vi "UHR-Fleezers Control (host) - 11.9.vi"() -> ()   [LabVIEW 2014] (continued)
        n2874 = Array Subset(array=w4167, index (col)=0 ("index"), length (col)=w4156) -> (w4166:dbl[][])  [unwired: 2 in]
        n2875 = Array Subset(array=w4167, index (col)=w4156) -> (w4164:dbl[][])  [unwired: 3 in]
        n2876 = Array Subset(array=w4241, index (col)=0 ("index"), length (col)=w4156) -> (w4240:dbl[][])  [unwired: 2 in]
        n2877 = Array Subset(array=w4241, index (col)=w4156) -> (w4238:dbl[][])  [unwired: 3 in]
        n2878 = Array Subset(array=w4224, index (col)=0 ("index"), length (col)=w4156) -> (w4229:dbl[][])  [unwired: 2 in]
        n2879 = Array Subset(array=w4224, index (col)=w4156) -> (w4227:dbl[][])  [unwired: 3 in]
        n2880 = for {
          tunnel: w4236 -> [w4278] mode=indexing
          tunnel: [w4277] -> w4235 mode=indexing
          workers-P: _ -> [_]
          n2881 = Reverse 1D Array(array=w4278) -> (reversed array=w4277:dbl[])
        }
        n2882 = for {
          tunnel: w4222 -> [w4274] mode=indexing
          tunnel: [w4273] -> w4221 mode=indexing
          workers-P: _ -> [_]
          n2883 = Reverse 1D Array(array=w4274) -> (reversed array=w4273:dbl[])
        }
        n2884 = for {
          tunnel: w4166 -> [w4272] mode=indexing
          tunnel: [w4271] -> w4165 mode=indexing
          workers-P: _ -> [_]
          n2885 = Reverse 1D Array(array=w4272) -> (reversed array=w4271:dbl[])
        }
        n2886 = for {
          tunnel: w4240 -> [w4280] mode=indexing
          tunnel: [w4279] -> w4239 mode=indexing
          workers-P: _ -> [_]
          n2887 = Reverse 1D Array(array=w4280) -> (reversed array=w4279:dbl[])
        }
        n2888 = for {
          tunnel: w4229 -> [w4276] mode=indexing
          tunnel: [w4275] -> w4228 mode=indexing
          workers-P: _ -> [_]
          n2889 = Reverse 1D Array(array=w4276) -> (reversed array=w4275:dbl[])
        }
        n2890 = Index Array(array=w4241, index (row)=0) -> (element=→"Waveform Graph":dbl[])  [unwired: 1 in]
        n2891 = Add(x=w4235, y=w4234) -> (x+y=w4233:dbl[][])
        n2892 = Add(x=w4221, y=w4220) -> (x+y=w4219:dbl[][])
        n2893 = Add(x=w4165, y=w4164) -> (x+y=w4149:dbl[][])
        n2894 = Add(x=w4239, y=w4238) -> (x+y=w4213:dbl[][])
        n2895 = Add(x=w4228, y=w4227) -> (x+y=w4226:dbl[][])
        n2896 = Divide(x=w4219, y=2) -> (x/y=w4217:dbl[][])
        n2897 = Divide(x=w4233, y=2) -> (x/y=w4178:dbl[][])
        n2898 = Divide(x=w4226, y=2) -> (x/y=w4180:dbl[][])
        n2899 = To Single Precision Float(number=w4213) -> (single precision float=w4212:sgl[][])
        n2900 = Transpose 2D Array(2D array=w4217) -> (transposed array=→"Data map":dbl[][])
        n2901 = To Single Precision Float(number=w4149) -> (single precision float=w4153:sgl[][])
        n2902 = To Single Precision Float(number=w4178) -> (single precision float=w4184:sgl[][])
        n2903 = To Single Precision Float(number=w4180) -> (single precision float=w4181:sgl[][])
        n2904 = call "IMAQ ArrayToImage"("Image Pixels (Float)"=w4212, "Image"=w4146) -> ("Image Out"=w4215:T2)  [unwired: 8 in, 1 out]
        n2905 = call "IMAQ ArrayToImage"("Image Pixels (Float)"=w4153, "Image"=w4145) -> ("Image Out"=w4155:T2)  [unwired: 8 in, 1 out]
        n2906 = call "IMAQ ArrayToImage"("Image Pixels (Float)"=w4184, "Image"=w4144) -> ("Image Out"=w4186:T2)  [unwired: 8 in, 1 out]
        n2907 = call "IMAQ ArrayToImage"("Image Pixels (Float)"=w4181, "Image"=w4143) -> ("Image Out"=w4183:T2)  [unwired: 8 in, 1 out]
        n2908 = call "IMAQ Symmetry"("Type of Symmetry"=w4214, "Image Src"=w4215) -> ("Image Dst Out"=w4210:T2)  [unwired: 3 in, 1 out]
        n2909 = call "IMAQ Symmetry"("Type of Symmetry"=w4154, "Image Src"=w4155) -> ("Image Dst Out"=w4151:T2)  [unwired: 3 in, 1 out]
        n2910 = call "IMAQ Symmetry"("Type of Symmetry"=w4185, "Image Src"=w4186) -> ("Image Dst Out"=→"Detection Laser X":T2)  [unwired: 3 in, 1 out]
        n2911 = call "IMAQ Symmetry"("Type of Symmetry"=w4182, "Image Src"=w4183) -> ("Image Dst Out"=→"Detection Laser Y":T2)  [unwired: 3 in, 1 out]
        n2912 = call "IMAQ Set Simple Calibration"("Calibration Axis Info"=T36 {"Origin Pixel"={"X"=0.0, "Y"=0.0}, "Angle Relative to Horizontal (deg)"=0.0, "Axis Reference"=0}, "Grid Descriptor"=T37 {"X Step"=0.3, "Y Step"=0.3, "Unit"=enum."Undefined"}, "Image"=w4210) -> ("Calibrated Image"=→"APD 1":T2)  [unwired: 7 in, 1 out]
        n2913 = call "IMAQ Set Simple Calibration"("Calibration Axis Info"=T36 {"Origin Pixel"={"X"=0.0, "Y"=0.0}, "Angle Relative to Horizontal (deg)"=0.0, "Axis Reference"=0}, "Grid Descriptor"=T37 {"X Step"=0.3, "Y Step"=0.3, "Unit"=enum."Undefined"}, "Image"=w4151) -> ("Calibrated Image"=→"APD 2":T2)  [unwired: 7 in, 1 out]
      }
    }
    n2914 = Subtract(x=w3595, y="APD 2 Offset") -> (x-y=w3592:waveform(dbl))
    n2915 = Subtract(x=w3597, y="APD 1 Offset") -> (x-y=w3593:waveform(dbl))
    n2916 = Index Array(array=w3612, index=3) -> (element=w3672:waveform(dbl))
    n2917 = Index Array(array=w3612, index=6) -> (element=w3669:waveform(dbl))
    n2918 = Build Array(w3593, w3592) -> (→"APD Chart":waveform(dbl)[])
    n2919 = Array Size(array=w3663) -> (size(s)=w3716:i32)
    n2920 = call <vilib>:"Std Deviation and Variance.vi"("X"=w3605) -> ("standard deviation"=w3604:dbl)  [unwired: 1 in, 2 out]
    n2921 = Add Array Elements(numeric array=w3605) -> (sum=w3607:u32)
    n2922 = Add Array Elements(numeric array=w3663) -> (sum=w3726:u32)
    n2923 = call <vilib>:"Std Deviation and Variance.vi"("X"=w3663) -> ("standard deviation"=w3662:dbl)  [unwired: 1 in, 2 out]
    n2924 = Divide(x="T1 offset_x (mV)", y=1000.0) -> (x/y=w3673:dbl)
    n2925 = Divide(x=w3604, y=w3603) -> (x/y=w3600:dbl)
    "Rate sigma (Hz) 2" <- w3600
    n2926 = Multiply(x=w3603, y=w3716) -> (x*y=w3606:dbl)
    "Int. Time (s)" <- w3606
    n2927 = Divide(x=w3607, y=w3606) -> (x/y=w3601:dbl)
    "APD 2 Rate (Hz)" <- w3601
    n2928 = Divide(x=w3726, y=w3606) -> (x/y=w3660:dbl)
    "APD 1 Rate (Hz)" <- w3660
    n2929 = Divide(x=w3662, y=w3603) -> (x/y=w3661:dbl)
    "Rate sigma (Hz)" <- w3661
    n2930 = Divide(x=w3600, y=w3601) -> (x/y=→"Sigma/Mean 2":dbl)
    n2931 = Divide(x=w3661, y=w3660) -> (x/y=→"s/Mean":dbl)
    n2932 = feedback-in #26("Calibration") -> ()
    n2933 = feedback #26(u16 1 ("Calibration")) -> (w3693:u16)
    n2934 = Divide(x="T2 offset_x (mV)", y=1000.0) -> (x/y=w3671:dbl)
    n2935 = case shown="0, Default" "Calibration" {
      tunnel: "T1 a_x (nm/V)" -> [_ w4109 w4130]
      tunnel: "T1 k_x (pN/nm)" -> [_ _ w4120]
      tunnel: "T2 a_x (nm/V)" -> [_ w4108 w4128]
      tunnel: "T2 k_x (pN/nm)" -> [_ _ w4121]
      tunnel: w3672 -> [w4091 w4106 w4126]
      tunnel: w3669 -> [w4090 w4104 w4124]
      tunnel: [w4091 w4103 w4123] -> w3702
      tunnel: [w4090 w4102 w4122] -> w3701
      tunnel: ["T1 X (V)" ("Label.Text") "T1 X (nm)" ("Label.Text") "T1 X (pN)" ("Label.Text")] -> w3690
      tunnel: ["T2 X (V)" ("Label.Text") "T2 X (nm)" ("Label.Text") "T2 X (pN)" ("Label.Text")] -> w3689
      tunnel: ["Position (V)" ("Label.Text") "Position (nm)" ("Label.Text") "Force (pN)" ("Label.Text")] -> w3691
      tunnel: w3671 -> [_ w4094 w4113]
      tunnel: w3673 -> [_ w4097 w4115]
      tunnel: ["Mean (V)" ("Label.Text") "Mean (nm)" ("Label.Text") "Mean (pN)" ("Label.Text")] -> w3686
      tunnel: ["Difference (V)" ("Label.Text") "Difference (nm)" ("Label.Text") "Difference (pN)" ("Label.Text")] -> w3620
      frame 0, Default {
      }
      frame 1 {
        n2936 = Unbundle By Name(w4106) -> ("Y"=w4110:dbl[])
        n2937 = Unbundle By Name(w4104) -> ("Y"=w4095:dbl[])
        n2938 = Subtract(x=w4110, y=w4097) -> (x-y=w4098:dbl[])
        n2939 = Subtract(x=w4095, y=w4094) -> (x-y=w4096:dbl[])
        n2940 = Multiply(x=w4096, y=w4108) -> (x*y=w4105:dbl[])
        n2941 = Multiply(x=w4109, y=w4098) -> (x*y=w4107:dbl[])
        n2942 = Bundle By Name(cluster=w4104, "Y"=w4105) -> (w4102:waveform(dbl))
        n2943 = Bundle By Name(cluster=w4106, "Y"=w4107) -> (w4103:waveform(dbl))
      }
      frame 2 {
        n2944 = Unbundle By Name(w4126) -> ("Y"=w4131:dbl[])
        n2945 = Unbundle By Name(w4124) -> ("Y"=w4129:dbl[])
        n2946 = Subtract(x=w4129, y=w4113) -> (x-y=w4114:dbl[])
        n2947 = Subtract(x=w4131, y=w4115) -> (x-y=w4116:dbl[])
        n2948 = Compound Arithmetic op=MULTIPLY(w4114, w4128, w4121) -> (w4125:dbl[])
        n2949 = Compound Arithmetic op=MULTIPLY(w4120, w4130, w4116) -> (w4127:dbl[])
        n2950 = Bundle By Name(cluster=w4124, "Y"=w4125) -> (w4122:waveform(dbl))
        n2951 = Bundle By Name(cluster=w4126, "Y"=w4127) -> (w4123:waveform(dbl))
      }
    }
    n2952 = Not Equal?(x=w3693, y="Calibration") -> (x != y?=w3650:bool)
    n2953 = case shown="True" w3650 {
      tunnel: w3691 -> [_ w4084]
      tunnel: w3690 -> [_ w4083]
      tunnel: w3689 -> [_ w4082]
      tunnel: w3686 -> [_ w4081]
      tunnel: w3620 -> [_ w4080]
      frame False {
      }
      frame True {
        n2954 = property on="Force" class="WFChart (strict)"("YScale.NameLbl.Text"=w4084) -> ()  [unwired: 2 in, 2 out]
        n2955 = property on="T2 X" class="DigNum (strict)"("Caption.Text"=w4082) -> ()  [unwired: 2 in, 2 out]
        n2956 = property on="T1 X" class="DigNum (strict)"("Caption.Text"=w4083) -> ()  [unwired: 2 in, 2 out]
        n2957 = property on="Mean" class="DigNum (strict)"("Caption.Text"=w4081) -> ()  [unwired: 2 in, 2 out]
        n2958 = property on="Difference" class="DigNum (strict)"("Caption.Text"=w4080) -> ()  [unwired: 2 in, 2 out]
      }
    }
    n2959 = Unbundle By Name(w3672) -> ("Y"=w3675:dbl[])
    n2960 = Unbundle By Name(w3669) -> ("Y"=w3678:dbl[])
    n2961 = Subtract(x=w3675, y=w3673) -> (x-y=w3676:dbl[])
    n2962 = Subtract(x=w3678, y=w3671) -> (x-y=w3677:dbl[])
    n2963 = Multiply(x=w3677, y="T2 a_x (nm/V)") -> (x*y=w3465:dbl[])
    n2964 = Multiply(x="T1 a_x (nm/V)", y=w3676) -> (x*y=w3466:dbl[])
    n2965 = Not(x="Trap Trig. Fl.") -> (.not. x?=w3502:bool)
    n2966 = Multiply(x=w3701, y=-1.0) -> (x*y=w3680:waveform(dbl))
    n2967 = Subtract(x=w3466, y=w3465) -> (x-y=w3668:dbl[])
    n2968 = Unbundle By Name(w3701) -> ("Y"=w3639:dbl[])
    n2969 = Unbundle By Name(w3702) -> ("Y"=w3467:dbl[])
    n2970 = Negate(x=w3668) -> (-x=w3463:dbl[])
    n2971 = Build Array(w3702, w3680) -> (→"Force":waveform(dbl)[])
    n2972 = Subtract(x=w3463, y="Offset (nm)") -> (x-y=w3637:dbl[])
    n2973 = case shown="True" "Read Lateness and Rel Phase" {
      tunnel: w3483 -> [w4057 w4079]
      tunnel: w3482 -> [w4058 w4078]
      tunnel: [w4057 w4077] -> w3666
      tunnel: [w4058 w4076] -> w3665
      frame False {
      }
      frame True {
        n2974 = xnode "Read/Write Control"("FPGA VI Reference In"=w4079, "error in"=w4078) -> ("FPGA VI Reference Out"=w4077:T19, "error out"=w4076:errorcluster, "GI Relative phase"=→"GI relative phase":i16, "Relative phase"=→"Relative phase (AI1)":i16, "AI Late Counter"=→"Late Counter (AI1)":u8, "GI Late Counter"=→"GI Late Counter":u8, "MCL Late Counter"=→"MCL Late Counter":u8, "MCL Relative Phase"=→"Relative Phase (MCL)":i16, "APD Acq Relative Phase"=→"APD Acq Relative Phase":i16, "APD 1 Gate Relative Phase"=→"APD 1 Gate Relative Phase":i16, "APD 2 Gate Relative Phase"=→"APD 2 Gate Relative Phase":i16, "APD Acq Late Counter"=→"APD Acq Late Counter":u8, "APD 1 Gate Late Counter"=→"APD 1 Gate Late Counter":u8, "APD 2 Gate Late Counter"=→"APD 2 Gate Late Counter":u8, "Green FB Relative Phase"=→"Relative phase (Green FB)":i16, "GI Relative phase 2"=→"GI relative phase 2":i16, "GI Late Counter 2"=→"GI Late Counter 2":u8, "Trap Pos FIFO Timeout"=→"Trap Pos FIFO Timeout":u16, "Trap AI FIFO Timeout"=→"Trap AI FIFO Timeout":u16)
      }
    }
    n2975 = call-poly <vilib>:"Mean.vi"("X"=w3639) -> ("mean"=w3469:dbl)  [unwired: 1 out]
    "T2 X" <- w3469
    n2976 = Negate(x=w3639) -> (-x=w3640:dbl[])
    n2977 = call-poly <vilib>:"Mean.vi"("X"=w3467) -> ("mean"=w3470:dbl)  [unwired: 1 out]
    "T1 X" <- w3470
    n2978 = Negate(x=w3469) -> (-x=w3468:dbl)
    n2979 = Bundle By Name(cluster=w3672, "Y"=w3637) -> (w3611:waveform(dbl))
    "Bead Separation" <- w3611
    n2980 = Add(x=w3467, y=w3640) -> (x+y=w3641:dbl[])
    n2981 = Add(x=w3470, y=w3468) -> (x+y=w3688:dbl)
    n2982 = Subtract(x=w3470, y=w3468) -> (x-y=→"Difference":dbl)
    n2983 = Divide(x=w3641, y=2.0) -> (x/y=→"Vec Mean of T1 T2":dbl[])
    n2984 = Divide(x=w3688, y=2.0) -> (x/y=w3643:dbl)
    "Mean" <- w3643
    n2985 = feedback-in #27("Trap Trig. Fl.") -> ()
    n2986 = feedback #27("Trap Trig. Fl.") -> (w3500:bool)
    n2987 = And(x=w3502, y=w3500) -> (x .and. y?=w3501:bool)
    n2988 = case "If have just turned off triggering" shown="True" w3501 {
      tunnel: w3483 -> [_ w3887]
      tunnel: w3482 -> [_ w3886]
      frame False {
      }
      frame True {
        w3885 = FALSE ("FPGA Trap Trig")
        n2989 = xnode "Read/Write Control"("FPGA VI Reference In"=w3887, "error in"=w3886, "FPGA Trap Trig"=w3885) -> ("FPGA VI Reference Out"=w3884:T19, "error out"=w3883:errorcluster)
        n2990 = xnode "Read/Write Control"("FPGA VI Reference In"=w3884, "error in"=w3883, "TTrig?"=w3885) -> ()  [unwired: 2 out]
        n2991 = local write "Initializing"(FALSE ("Initializing")) -> ()
        n2992 = local write "Triggered"(FALSE ("Triggered")) -> ()
        n2993 = local write "Waiting"(FALSE ("Waiting")) -> ()
      }
    }
    n2994 = Not(x=w3500) -> (.not. x?=w3513:bool)
    n2995 = And(x="Trap Trig. Fl.", y=w3513) -> (x .and. y?=w3510:bool)
    n2996 = local read "Tether"() -> (w3644:bool)
    n2997 = Or(x=w3510, y="Reinitialize") -> (x .or. y?=w3496:bool)
    n2998 = feedback #28(w3506) -> (w3511:string)
    n2999 = Select(t=w3506, s=w3510, f=w3511) -> (s? t:f=w3505:string)
    n3000 = Select(t=w3506, s="Reinitialize", f=w3505) -> (s? t:f=w3504:string)
    n3001 = feedback #29(0) -> (w3508:i32)
    n3002 = feedback #30(w3637) -> (w3636:dbl[])
    n3003 = Build Array (concatenate)(w3637, w3636) -> (w3464:dbl[])
    n3004 = case "For determining if there is a tether still" shown="True" w3644 {
      tunnel: w3643 -> [_ w4011]
      frame False {
      }
      frame True {
        n3005 = Greater?(x="Lost Tether Alarm Threshold (pN)", y=w4011) -> (0:w4009:bool)
        n3006 = case shown="True" w4009 {
          frame False {
          }
          frame True {
            w4012 = TRUE
            w4016 = FALSE ("Multiple tether")
            w4017 = FALSE ("Value (Signaling)")
            n3007 = flat-sequence {
              frame #0 {
                # "stop only if saving"
                n3008 = local read "Saving..."() -> (w4029:bool)
                n3009 = And(x=w4029, y="TA Cancel Save?") -> (x .and. y?=w4028:bool)
                n3010 = local write "Stop Saving"(w4028) -> ()
              }
              frame #1 {
                n3011 = case shown="True" "TA Green Off?" {
                  frame False {
                  }
                  frame True {
                    w4032 = FALSE ("Fl. Triggered...")
                    n3012 = local write "Fl. Triggered..."(w4032) -> ()
                    n3013 = property on="Green ON/Interlacing" class="Bool (strict)"("Val(Sgnl)"=w4032) -> ()  [unwired: 2 in, 2 out]
                  }
                }
              }
            }
            n3014 = local read "Time tether formed"() -> (w4023:timestamp)
            n3015 = Get Date/Time In Seconds() -> (seconds since 1Jan1904=w4024:timestamp)
            n3016 = Subtract(x=w4024, y=w4023) -> (x-y=w4022:dbl)
            n3017 = Number To Decimal String(number=w4022) -> (decimal integer string=w4019:string)  [unwired: 1 out]
            n3018 = local read "Messages"() -> (w4026:string)
            n3019 = call <vilib>:"Beep.vi"("use system alert? (T)"=FALSE, "duration (msec)"=u32 200, "frequency (Hz)"=u32 200) -> ()  [unwired: 9 out]
            n3020 = Concatenate Strings("Lost tether (" ("Message to add"), w4019, " s)." ("string")) -> (w4021:string)
            n3021 = local write "Tether"(FALSE ("Tether")) -> ()
            n3022 = call "Update messages.vi"("Message to add"=w4021, "Old message string"=w4026) -> ("New message string"=w4025:string)
            n3023 = local write "Messages"(w4025) -> ()
            n3024 = local write "Pause dwell"(w4017) -> ()
            n3025 = property on="Fl. Triggered..." class="Bool (strict)"("Val(Sgnl)"=w4017) -> ()  [unwired: 2 in, 2 out]
            n3026 = local write "Dip for Protein"(w4017) -> ()
            n3027 = property on="Trap Pos. FB ON" class="Bool (strict)"("Val(Sgnl)"=w4017) -> ()  [unwired: 2 in, 2 out]
            n3028 = property on="Trap Trig. Fl." class="Bool (strict)"("Val(Sgnl)"=w4017) -> ()  [unwired: 2 in, 2 out]
            n3029 = local write "Multiple tether"(w4016) -> ()
            n3030 = local write "Bad fit"(w4016) -> ()
            n3031 = local write "Hysteresis"(w4016) -> ()
            n3032 = local write "Good tether"(w4016) -> ()
            n3033 = local write "Save scans"(w4012) -> ()
            n3034 = local write "Restart DMA? (AOD)"(w4012) -> ()
          }
        }
      }
    }
    n3035 = case "For triggering actions based on the trap position (e.g., turning the excitation laser on if trap under feedback moves so far)" shown="True" "Trap Trig. Fl." {
      tunnel: w3491 -> [_ w3900]
      tunnel: w3504 -> [_ w3899]
      tunnel: ["" ("t") w3898] -> w3512
      tunnel: w3496 -> [_ w3897]
      tunnel: [0 ("t") w3896] -> w3509
      tunnel: w3508 -> [_ w3895]
      tunnel: w3483 -> [_ w3894]
      tunnel: w3482 -> [_ w3893]
      frame False {
      }
      frame True {
        n3036 = case shown="\"Wait for trigger\"" w3899 {
          tunnel: w3900 -> [w3917 _ _ w3965]
          tunnel: [w3914 w3946 "" ("t") w3968] -> w3898
          tunnel: w3897 -> [_ _ _ w3956]
          tunnel: [w3913 w3943 0 ("t") w3957] -> w3896
          tunnel: w3895 -> [_ w3945 _ w3963]
          tunnel: w3894 -> [w3902 w3940 _ w3959]
          tunnel: w3893 -> [w3901 w3939 _ w3958]
          frame "Wait for trigger" {
            n3037 = local read "Trap Trig. (FPGA)"() -> (w3905:bool)
            n3038 = Subtract(x=w3917, y="Mean T1 Position\nto compare (nm)") -> (x-y=w3910:dbl[])
            n3039 = call <vilib>:"Std Deviation and Variance.vi"("X"=w3910) -> ("mean"=→"mean":dbl, "standard deviation"=→"standard\ndeviation":dbl)  [unwired: 1 in, 1 out]
            n3040 = Array Max & Min(array=w3910) -> (max value=→"max value":dbl, min value=→"min value":dbl)  [unwired: 2 out]
            n3041 = Greater?(x=w3910, y="Threshold (nm)") -> (0:w3920:bool[])
            n3042 = case shown="True" w3905 {
              tunnel: w3902 -> [_ w3926]
              tunnel: w3901 -> [_ w3925]
              tunnel: [FALSE ("TTrig?") w3924] -> w3908
              frame False {
              }
              frame True {
                n3043 = xnode "Read/Write Control"("FPGA VI Reference In"=w3926, "error in"=w3925) -> ("TTrig?"=w3924:bool)  [unwired: 2 out]
              }
            }
            n3044 = Or Array Elements(Boolean array=w3920) -> (logical OR=w3907:bool)
            n3045 = Select(t=w3908, s=w3905, f=w3907) -> (s? t:f=w3906:bool)
            n3046 = Not(x=w3905) -> (.not. x?=w3904:bool)
            n3047 = And(x=w3906, y=w3904) -> (x .and. y?=w3903:bool)
            n3048 = Select(t="Triggered", s=w3906, f="Wait for trigger") -> (s? t:f=w3914:string)
            n3049 = case shown="True" w3906 {
              tunnel: [0 0] -> w3913
              tunnel: w3902 -> [_ w3931]
              tunnel: w3901 -> [_ w3930]
              frame False {
                "Waiting" <- TRUE ("Waiting")
              }
              frame True {
                n3050 = xnode "Read/Write Control"("FPGA VI Reference In"=w3931, "error in"=w3930, "TTrig?"=FALSE) -> ()  [unwired: 2 out]
                n3051 = local read "Messages"() -> (w3934:string)
                n3052 = call <vilib>:"Beep.vi"() -> ()  [unwired: 12 in]
                n3053 = call "Update messages.vi"("Message to add"="Unwinding trigger.", "Old message string"=w3934) -> ("New message string"=w3935:string)
                n3054 = local write "Messages"(w3935) -> ()
                n3055 = local write "Waiting"(FALSE ("Waiting")) -> ()
                "Triggered" <- TRUE ("Triggered")
              }
            }
            n3056 = case "Only need to turn on laser if host triggered" shown="True" w3903 {
              frame False {
              }
              frame True {
                n3057 = property on="Green ON/Interlacing" class="Bool (strict)"("Val(Sgnl)"=TRUE ("Value (Signaling)")) -> ()  [unwired: 2 in, 2 out]
              }
            }
          }
          frame "Triggered" {
            n3058 = local read "Trap Trig. (FPGA)"() -> (w3942:bool)
            n3059 = Increment(x=w3945) -> (x+1=w3943:i32)
            n3060 = Greater Or Equal?(x=w3943, y="Fl. ON time (n)") -> (x >= y?=w3941:bool)
            n3061 = Select(t="Wait for trigger", s=w3941, f="Triggered" ("t")) -> (s? t:f=w3946:string)
            n3062 = And(x=w3941, y=w3942) -> (x .and. y?=w3938:bool)
            n3063 = case shown="True" w3938 {
              tunnel: w3940 -> [_ w3950]
              tunnel: w3939 -> [_ w3949]
              frame False {
              }
              frame True {
                n3064 = xnode "Read/Write Control"("FPGA VI Reference In"=w3950, "error in"=w3949, "FPGA Trap Trig"=TRUE) -> ()  [unwired: 2 out]
              }
            }
            n3065 = case shown="True" w3941 {
              frame False {
              }
              frame True {
                w3952 = FALSE ("Value (Signaling)")
                n3066 = local write "Triggered"(w3952) -> ()
                n3067 = local write "Waiting"(TRUE ("Waiting")) -> ()
                n3068 = property on="Green ON/Interlacing" class="Bool (strict)"("Val(Sgnl)"=w3952) -> ()  [unwired: 2 in, 2 out]
              }
            }
          }
          frame "Do nothing" {
          }
          frame "Initialize", Default {
            n3069 = Increment(x=w3963) -> (x+1=w3967:i32)
            n3070 = Select(t=1, s=w3956, f=w3967) -> (s? t:f=w3957:i32)
            n3071 = feedback #31(w3965) -> (w3971:dbl[])
            n3072 = Build Array (concatenate)(w3965, w3971) -> (w3964:dbl[])
            n3073 = Greater Or Equal?(x=w3957, y="Wait to get offset (n)") -> (x >= y?=w3960:bool)
            n3074 = Select(t=w3965, s=w3956, f=w3964) -> (s? t:f=w3966:dbl[])
            n3075 = feedback-in #31(w3966) -> ()
            n3076 = call-poly <vilib>:"Mean.vi"("X"=w3966) -> ("mean"=w3961:dbl)  [unwired: 1 out]
            n3077 = local write "Mean T1 Position\nto compare (nm)"(w3961) -> ()
            n3078 = case shown="True" w3956 {
              tunnel: w3959 -> [_ w3977]
              tunnel: w3958 -> [_ w3976]
              frame False {
              }
              frame True {
                w3973 = FALSE ("FPGA Trap Trig")
                n3079 = xnode "Read/Write Control"("FPGA VI Reference In"=w3977, "error in"=w3976, "FPGA Trap Trig"=w3973) -> ("FPGA VI Reference Out"=w3975:T19, "error out"=w3974:errorcluster)
                n3080 = xnode "Read/Write Control"("FPGA VI Reference In"=w3975, "error in"=w3974, "TTrig?"=w3973) -> ()  [unwired: 2 out]
              }
            }
            n3081 = Select(t="Wait for trigger", s=w3960, f="Initialize") -> (s? t:f=w3968:string)
            n3082 = case shown="True" w3960 {
              tunnel: w3961 -> [_ w3980]
              tunnel: w3959 -> [_ w3989]
              tunnel: w3958 -> [_ w3988]
              frame False {
                n3083 = local write "Waiting"(FALSE ("Waiting")) -> ()
                "Initializing" <- TRUE ("Initializing")
              }
              frame True {
                n3084 = local read "Threshold (nm)"() -> (w3992:dbl)
                n3085 = local read "AOM X Cal (nm/MHz)"() -> (w3991:dbl)
                n3086 = Add(x=w3980, y=w3992) -> (x+y=w3993:dbl)
                n3087 = Divide(x=w3993, y=w3991) -> (x/y=w3990:dbl)
                n3088 = call "IR AOM freq to word.vi"("Frequency In (MHz)"=w3990) -> ("Frequency Word Out (double)"=w3987:dbl)
                n3089 = local write "Initializing"(FALSE ("Initializing")) -> ()
                n3090 = local write "Waiting"(TRUE ("Waiting")) -> ()
                n3091 = To Quad Integer(1:w3987) -> (0:w3986:i64)
                n3092 = xnode "Read/Write Control"("FPGA VI Reference In"=w3989, "error in"=w3988, "FPGA TTrig Thresh"=w3986) -> ("FPGA VI Reference Out"=w3983:T19, "error out"=w3982:errorcluster)
                n3093 = xnode "Read/Write Control"("FPGA VI Reference In"=w3983, "error in"=w3982, "FPGA Trap Trig"=TRUE) -> ()  [unwired: 2 out]
              }
            }
          }
        }
      }
    }
    n3094 = feedback-in #28(w3512) -> ()
    n3095 = feedback-in #29(w3509) -> ()
    n3096 = Split 1D Array(array=w3464, index=w3526) -> (first subarray=w3633:dbl[])  [unwired: 1 out]
    n3097 = feedback-in #30(w3633) -> ()
    n3098 = call-poly <vilib>:"Mean.vi"("X"=w3633) -> ("mean"=w3632:dbl)  [unwired: 1 out]
    "Bead Mean (nm)" <- w3632
    n3099 = Subtract(x=w3633, y=w3632) -> (x-y=w3631:dbl[])
    n3100 = Square(x=w3631) -> (x^2=w3630:dbl[])
    n3101 = call-poly <vilib>:"Mean.vi"("X"=w3630) -> ("mean"=w3629:dbl)  [unwired: 1 out]
    n3102 = Square Root(x=w3629) -> (sqrt(x)=w3628:dbl)
    n3103 = Multiply(x=10.0, y=w3628) -> (x*y=→"RMS (Å)":dbl)
    n3104 = xnode ("Read/Write Control")("FPGA VI Reference In"=w3666, "error in"=w3665) -> ("FPGA VI Reference Out"=w3494:T19, "error out"=w3493:errorcluster, "AI2 Y Sum Set 1"=w3770:i16, "AI2 Y Sum Set 2"=w3769:i16, "AI1 X Set 1"=w3557:fxp<+/-,16,1>, "AI1 X Set 2"=w3556:fxp<+/-,16,1>, "Trap Pos FB Int Signal"=→"Trap Pos FB Int Signal":fxp<+/-,24,9>, "Trap Pos FB Int-Norm Signal"=→"Trap Pos FB Int-Norm Signal":fxp<+/-,16,1>, "Trap Pos FB Action"=w3550:i64, "Scanning"=→"AOD Scanning":bool, "Scan I"=→"AOD Scan I":u64, "Scanning MCL"=w3772:bool, "Scan I (MCL)"=→"MCL Scan I":u64, "Green FB Signals"=w3711:T47, "Trap Pos FB Action"=w3481:i64, "Wiggling 1"=→"Wiggling T1":bool, "TTrig Fin Thresh"=w3477:i64, "Wiggling 2"=→"Wiggling T2":bool)  [unwired: 2 out]
    "MCL Scanning" <- w3772
    "Trap Pos FB Action" <- w3550
    n3105 = local read "FB Trig Integrate"() -> (w3475:u32)
    n3106 = Divide(x=w3481, y=w3475) -> (x/y=w3474:dbl)
    "TTrig Sig (Int)" <- w3474
    n3107 = Divide(x=w3477, y=w3475) -> (x/y=w3472:dbl)
    "TTrig Fin Thresh (Int)" <- w3472
    n3108 = local read "AOM X Cal (nm/MHz)"() -> (w3480:dbl)
    n3109 = local read "AI2 (V)"() -> (w3771:cluster{"Set 1":dbl, "Set 2":dbl})
    n3110 = Bundle By Name(cluster=w3771, "Set 1"=w3770, "Set 2"=w3769) -> (w3767:cluster{"Set 1":dbl, "Set 2":dbl})
    n3111 = Divide(x=w3550, y=327.67) -> (x/y=w3459:dbl)
    n3112 = local read "Trap X (AI1)"() -> (w3570:T10)
    n3113 = call "IR AOM word double to freq.vi"("Frequency Word In (double)"=w3472) -> ("Frequency Out (MHz)"=w3471:dbl)
    n3114 = call "IR AOM word double to freq.vi"("Frequency Word In (double)"=w3474) -> ("Frequency Out (MHz)"=w3473:dbl)
    n3115 = Divide(x=w3767, y=3276.7) -> (x/y=w3766:cluster{"Set 1":dbl, "Set 2":dbl})
    n3116 = Multiply(x=w3473, y=w3480) -> (x*y=w3479:dbl)
    "TTrig Sig (nm)" <- w3479
    n3117 = Multiply(x=w3471, y=w3480) -> (x*y=w3478:dbl)
    "TTrig Fin Thresh (nm)" <- w3478
    n3118 = local write "AI2 (V)"(w3766) -> ()
    n3119 = local read "Trap Pos. FB Range"() -> (w3458:T12)
    n3120 = Bundle(cluster=w3570, "Trap 1"=w3557, "Trap 2"=w3556) -> (→"Trap X (AI1)":T10)
    n3121 = Bundle(w3479, w3478) -> (→"TTrig":cluster{dbl, dbl})  [unwired: 1 in]
    n3122 = Unbundle(w3458) -> ("output high"=w3457:fxp<+/-,64,32>)  [unwired: 1 out]
    n3123 = Divide(x=w3459, y=w3457) -> (x/y=→"Action (%)":dbl)
    n3124 = Divide(x=w3711, y=3276.7) -> (x/y=w3707:T48)
    n3125 = Unbundle By Name(w3707) -> ("Green FB Ch 0"=w3710:dbl, "Green FB Ch 1"=w3709:dbl, "Green FB Ch 2"=w3708:dbl)
    n3126 = Divide(x=w3710, y=w3708) -> (x/y=w3706:dbl)
    n3127 = Divide(x=w3709, y=w3708) -> (x/y=w3705:dbl)
    n3128 = flat-sequence "To save data" {
      tunnel: [w4853] -> w3790
      tunnel: [w4854] -> w3789
      tunnel: w3742 -> [w4826]
      tunnel: w3499 -> [w4851]
      tunnel: ["Save Calibration"] -> w3763
      tunnel: w3760 -> [w4850]
      tunnel: [w4844] -> w3759
      tunnel: [w4841] -> w3758
      tunnel: [w4838] -> w3757
      tunnel: w3741 -> [w4840]
      tunnel: w3648 -> [w4834]
      tunnel: [w4834] -> w3647
      tunnel: ["Start Saving"] -> w3613
      tunnel: [w4828] -> w3539
      tunnel: [w4827] -> w3538
      tunnel: w3790 -> [w5093]
      tunnel: w3789 -> [w5092]
      tunnel: w3540 -> [w5091]
      tunnel: w3763 -> [w5090]
      tunnel: w3759 -> [w5088]
      tunnel: w3758 -> [w5087]
      tunnel: w3757 -> [w5086]
      tunnel: w3622 -> [w5085]
      tunnel: w3658 -> [w5084]
      tunnel: w3647 -> [w5083]
      tunnel: w3613 -> [w5082]
      tunnel: w3611 -> [w5081]
      tunnel: w3587 -> [w5080]
      tunnel: w3539 -> [w5079]
      tunnel: w3538 -> [w5078]
      tunnel: w3537 -> [w5077]
      tunnel: w3460 -> [w5076]
      frame #0 {
        n3129 = Or(x="Save N Sets", y="Start Saving") -> (x .or. y?=w4835:bool)
        n3130 = To Double Precision Float(number=w4850) -> (double precision float=w4845:dbl)
        n3131 = Build Array(w4835, "Save Calibration", w4826, w4840) -> (w4849:bool[])
        n3132 = Compound Arithmetic op=OR("Save Calibration", w4826, w4835, w4840) -> (w4852:bool)
        n3133 = Boolean Array To Number(Boolean array=w4849) -> (number=w4847:u32)
        n3134 = feedback #32(FALSE ("Save APD Data\nwith Trap Data")) -> (w4829:bool)
        n3135 = feedback #33(refnum<k0> refnum) -> (w4855:refnum<file>)
        n3136 = feedback #34(refnum<k0> refnum) -> (w4831:refnum<file>)
        n3137 = feedback #35(FALSE ("Save APD Data\nwith Trap Data")) -> (w4839:bool)
        n3138 = feedback #36(refnum<k0> refnum) -> (w4842:refnum<file>)
        n3139 = feedback #37(0) -> (w4857:i32)
        n3140 = feedback #38() -> (w4846:u32)  [unwired: 1 out]
        n3141 = case shown="True" w4852 {
          tunnel: [w4864 1] -> w4853
          tunnel: w4857 -> [w4866 _]
          tunnel: [w4865 w4884] -> w4854
          tunnel: w4855 -> [w4865 _]
          tunnel: w4851 -> [_ w4904]
          tunnel: w4845 -> [_ w4902]
          tunnel: w4847 -> [_ w4905]
          tunnel: [w4863 w4883] -> w4844
          tunnel: w4846 -> [w4863 _]
          tunnel: [w4862 w4881] -> w4841
          tunnel: w4842 -> [w4862 _]
          tunnel: [w4861 w4880] -> w4838
          tunnel: w4839 -> [w4861 _]
          tunnel: "Start Saving" -> [_ w4878]
          tunnel: w4834 -> [_ w4877]
          tunnel: [w4860 w4868] -> w4827
          tunnel: w4831 -> [w4860 _]
          tunnel: [w4859 w4867] -> w4828
          tunnel: w4829 -> [w4859 _]
          frame False {
            n3142 = Increment(x=w4866) -> (x+1=w4864:i32)
          }
          frame True {
            w4874 = FALSE ("Start Saving")
            w4879 = 9.0  # File Version
            w4887 = FALSE ("prepend array or string size? (T)")
            w4885 = T24."big-endian, network order" ("byte order (0:big-endian, network order)")
            n3143 = local read "BD 1 Frequency 1 (MHz)"() -> (w4901:dbl)
            n3144 = local read "BD 2 Frequency 1 (MHz)"() -> (w4900:dbl)
            n3145 = local read "BD 1 Frequency 2 (MHz)"() -> (w4899:dbl)
            n3146 = local read "BD 2 Frequency 2 (MHz)"() -> (w4898:dbl)
            n3147 = local read "BD 1 Frequency 3 (MHz)"() -> (w4897:dbl)
            n3148 = local read "BD 2 Frequency 3 (MHz)"() -> (w4896:dbl)
            n3149 = Array Size(array=w4877) -> (size(s)=w4876:i32)
            n3150 = To Double Precision Float(number=w4876) -> (double precision float=w4875:dbl)
            n3151 = local write "Save Calibration"(w4874) -> ()
            n3152 = local write "Start Saving"(w4874) -> ()
            n3153 = Build Array("Save APD Data\nwith Trap Data", "Save Trap Pos. Data") -> (w4871:bool[])
            n3154 = Boolean Array To Number(Boolean array=w4871) -> (number=w4870:u32)
            n3155 = Build Array(w4901, w4900, w4899, w4898, w4897, w4896) -> (w4895:dbl[])
            n3156 = case shown="1, Default" w4905 {
              tunnel: w4904 -> [w4978 w5000 w5016 w5054]
              tunnel: w4875 -> [w4983 w5007 w5036 w5073]
              tunnel: w4902 -> [w4982 w5006 w5035 w5072]
              tunnel: [w4979 w5002 w5027 w5064] -> w4893
              tunnel: [w4971 "Cal sets to save" w5017 w5055] -> w4883
              tunnel: w4895 -> [w4980 w5003 w5029 w5066]
              tunnel: "Save APD Data\nwith Trap Data" -> [w4977 _ w5013 w5052]
              tunnel: [w4977 FALSE ("Save APD Data\nwith Trap Data") w5013 w5052] -> w4880
              tunnel: w4879 -> [w4974 w4997 w5011 w5050]
              tunnel: w4878 -> [w4973 _ _ _]
              tunnel: [w4965 "Active cal?" w5010 w5040] -> w4867
              tunnel: "Save Trap Pos. Data" -> [w4965 _ w5010 w5040]
              tunnel: w4870 -> [w4964 _ w5009 w5039]
              frame 1, Default {
                # "timeseries"
                n3157 = case shown="True" "Profile" {
                  tunnel: [w4986 w4990] -> w4969
                  tunnel: [w4986 w4989] -> w4968
                  tunnel: [w4986 w4988] -> w4967
                  tunnel: [w4986 w4987] -> w4966
                  frame False {
                    w4986 = 0.0 ("f")
                  }
                  frame True {
                    n3158 = local read "Current Position"() -> (w4991:cluster{dbl, dbl, dbl})
                    n3159 = local read "Y change (mm)"() -> (w4987:dbl)
                    n3160 = Unbundle(w4991) -> (w4990:dbl, w4989:dbl, w4988:dbl)
                  }
                }
                n3161 = local read "Save ave N"() -> (w4985:dbl)
                n3162 = Multiply(x=w4985, y=w4978) -> (x*y=w4984:dbl)
                n3163 = To Double Precision Float(number=w4964) -> (double precision float=w4976:dbl)
                n3164 = Select(t=4.0, s="Profile", f=0.0) -> (s? t:f=w4960:dbl)
                n3165 = Build Array(w4974, w4978, w4984, w4983, w4982, w4960) -> (w4981:dbl[])
                n3166 = Build Array(w4976, w4969, w4968, w4967, w4966) -> (w4975:dbl[])
                n3167 = Select(t=u32 4000000000, s=w4973, f="N sets to save") -> (s? t:f=w4971:u32)
                n3168 = Build Array (concatenate)(w4981, w4980, w4975) -> (w4979:dbl[])
              }
              frame 2 {
                w4999 = 0.0 ("f")
                # "If doing active calibration,\nalso save trap position file"
                # "calibration"
                n3169 = property on="Wiggle" class="Bool (strict)"("Val(Sgnl)"="Active cal?") -> ()  [unwired: 2 in, 2 out]
                n3170 = Select(t=2.0, s="Active cal?", f=0.0) -> (s? t:f=w4993:dbl)
                n3171 = Build Array(w4993, w4999, w4999, w4999, w4999) -> (w4998:dbl[])
                n3172 = Build Array(w4997, w5000, w5000, w5007, w5006, 1.0 ("t")) -> (w5004:dbl[])
                n3173 = Build Array (concatenate)(w5004, w5003, w4998) -> (w5002:dbl[])
                "Calibrating..." <- TRUE ("Calibrating...")
              }
              frame 4 {
                w5014 = 0.0 ("f")
                # "scan dir (x/y = 0/1)"
                # "cycles/step"
                # "n scans (f/b)"
                # "steps"
                # "freq. range"
                # "AOD raster scan"
                n3174 = local read "Number of F/B Scans (AOD)"() -> (w5021:u16)
                n3175 = local read "Cycles/step (AOD)"() -> (w5023:u64)
                n3176 = local read "Scan Range (MHz)"() -> (w5026:dbl)
                n3177 = local read "Scan steps (AOD)"() -> (w5025:u64)
                n3178 = local read "Scan BD"() -> (w5033:bool)
                n3179 = local read "Save ave N"() -> (w5038:dbl)
                n3180 = Boolean To (0,1)(Boolean=w5033) -> (0, 1=w5032:i16)
                n3181 = To Double Precision Float(number=w5021) -> (double precision float=w5020:dbl)
                n3182 = To Double Precision Float(number=w5025) -> (double precision float=w5024:dbl)
                n3183 = To Double Precision Float(number=w5023) -> (double precision float=w5022:dbl)
                n3184 = To Double Precision Float(number=w5032) -> (double precision float=w5031:dbl)
                n3185 = Multiply(x=w5038, y=w5016) -> (x*y=w5037:dbl)
                n3186 = To Double Precision Float(number=w5009) -> (double precision float=w5015:dbl)
                n3187 = Build Array(w5015, w5014, w5014, w5014, w5014) -> (w5012:dbl[])
                n3188 = local read "N sets should be saved"() -> (w5018:dbl)
                n3189 = Build Array(w5031, w5026, w5024, w5022, w5020) -> (w5028:dbl[])
                n3190 = Build Array(w5011, w5016, w5037, w5036, w5035, 2.0 ("t")) -> (w5030:dbl[])
                n3191 = Round Toward +Infinity(x=w5018) -> (ceil(x): smallest int >= x=w5019:dbl)
                n3192 = Build Array (concatenate)(w5030, w5029, w5012, w5028) -> (w5027:dbl[])
                n3193 = To Unsigned Long Integer(number=w5019) -> (unsigned 32bit integer=w5017:u32)
              }
              frame 8 {
                w5047 = 0.0 ("f")
                # "MCL raster scan"
                n3194 = local read "Number of scans (MCL)"() -> (w5042:u64)
                n3195 = local read "Scan lines (y)"() -> (w5041:u64)
                n3196 = local read "2D or 1D Scan"() -> (w5044:bool)
                n3197 = local read "Scan Range (V)\n(of steps)"() -> (w5063:dbl)
                n3198 = local read "Fast Scan Dir"() -> (w5070:bool)
                n3199 = local read "Cycles/step (MCL)"() -> (w5060:u64)
                n3200 = local read "Scan steps (MCL)"() -> (w5062:u64)
                n3201 = Select(t=w5041, s=w5044, f=w5042) -> (s? t:f=w5043:u64)
                n3202 = Boolean To (0,1)(Boolean=w5044) -> (0, 1=w5046:i16)
                n3203 = local read "Save ave N"() -> (w5075:dbl)
                n3204 = local read "Initial X"() -> (w5049:dbl)
                n3205 = local read "Initial Y"() -> (w5048:dbl)
                n3206 = To Double Precision Float(number=w5046) -> (double precision float=w5045:dbl)
                n3207 = Boolean To (0,1)(Boolean=w5070) -> (0, 1=w5069:i16)
                n3208 = To Double Precision Float(number=w5043) -> (double precision float=w5058:dbl)
                n3209 = To Double Precision Float(number=w5062) -> (double precision float=w5061:dbl)
                n3210 = To Double Precision Float(number=w5060) -> (double precision float=w5059:dbl)
                n3211 = To Double Precision Float(number=w5069) -> (double precision float=w5068:dbl)
                n3212 = Multiply(x=w5075, y=w5054) -> (x*y=w5074:dbl)
                n3213 = To Double Precision Float(number=w5039) -> (double precision float=w5053:dbl)
                n3214 = local read "N sets should be saved (MCL)"() -> (w5056:dbl)
                n3215 = Build Array(w5053, w5045, w5047, w5047, w5047) -> (w5051:dbl[])
                n3216 = Build Array(w5068, w5063, w5061, w5059, w5058, w5049, w5048) -> (w5065:dbl[])
                n3217 = Build Array(w5050, w5054, w5074, w5073, w5072, 3.0 ("t")) -> (w5067:dbl[])
                n3218 = Round Toward +Infinity(x=w5056) -> (ceil(x): smallest int >= x=w5057:dbl)
                n3219 = Build Array (concatenate)(w5067, w5066, w5051, w5065) -> (w5064:dbl[])
                n3220 = To Unsigned Long Integer(number=w5057) -> (unsigned 32bit integer=w5055:u32)
              }
            }
            n3221 = local read "Index"() -> (w4910:dbl)
            n3222 = call "Create new save file.vi"("Insert"="", "Ext"=".dat", "Index In"=w4910) -> ("Path Out"=w4869:path, "Index Out"=w4882:dbl)
            n3223 = local write "Save file name"(w4869) -> ()
            n3224 = local write "Index"(w4882) -> ()
            n3225 = local write "Save index"(w4882) -> ()
            n3226 = Array Size(array=w4893) -> (size(s)=w4894:i32)
            n3227 = Open/Create/Replace File(file path (use dialog)=w4869, operation (0:open)=T25."create", access (0:read/write)=enum16{"read/write", "read-only", "write-only"}."write-only") -> (refnum out=w4907:refnum<file>)  [unwired: 1 in, 4 out]
            n3228 = local write "Saving..."(TRUE ("Saving...")) -> ()
            n3229 = To Double Precision Float(number=w4894) -> (double precision float=w4892:dbl)
            n3230 = String Length(string="Comment (data description)") -> (length=w4890:i32)
            n3231 = To Double Precision Float(number=w4890) -> (double precision float=w4889:dbl)
            n3232 = Deny Access(7:w4907) -> (3:w4906:refnum<file>)  [unwired: 1 in, 2 out]
            n3233 = Build Array (concatenate)(w4892, w4893, w4889) -> (w4891:dbl[])
            n3234 = case "If fluorescence data to be saved" shown="True" w4880 {
              tunnel: w4869 -> [_ w4959]
              tunnel: [refnum<k0> refnum w4939] -> w4881
              frame False {
              }
              frame True {
                w4938 = 0.0
                n3235 = local read "APD Integration Time (s)"() -> (w4944:dbl)
                n3236 = local read "N APD Samp/step"() -> (w4937:dbl)
                n3237 = Path To String(path=w4959) -> (string=w4958:string)
                n3238 = String Length(string=w4958) -> (length=w4957:i32)
                n3239 = Subtract(x=w4957, y=4) -> (x-y=w4955:i32)
                n3240 = String Subset(string=w4958, length (rest)=w4955) -> (substring=w4954:string)  [unwired: 1 out]
                n3241 = Build Array(w4944, w4937, w4938, w4938, w4938, w4938, w4938, w4938) -> (w4941:dbl[])
                n3242 = Concatenate Strings(w4954, "_fl.dat" ("string")) -> (w4952:string)
                n3243 = Array Size(array=w4941) -> (size(s)=w4943:i32)
                n3244 = String To Path(string=w4952) -> (path=w4948:path)
                n3245 = Open/Create/Replace File(file path (use dialog)=w4948, operation (0:open)=T25."create", access (0:read/write)=enum16{"read/write", "read-only", "write-only"}."write-only") -> (refnum out=w4949:refnum<file>)  [unwired: 1 in, 4 out]
                n3246 = Deny Access(7:w4949) -> (3:w4945:refnum<file>)  [unwired: 1 in, 2 out]
                n3247 = To Double Precision Float(number=w4943) -> (double precision float=w4942:dbl)
                n3248 = Build Array (concatenate)(w4942, w4941) -> (w4940:dbl[])
                n3249 = Write to Binary File(file (use dialog)=w4945, data=w4940, 5:FALSE ("prepend array or string size? (T)"), 9:T24."big-endian, network order" ("byte order (0:big-endian, network order)")) -> (refnum out=w4939:refnum<file>)  [unwired: 1 in, 3 out]
              }
            }
            n3250 = case shown="True" w4867 {
              tunnel: w4869 -> [_ w4921]
              tunnel: [refnum<k0> refnum w4920] -> w4868
              frame False {
              }
              frame True {
                w4916 = 0.0 ("element")
                n3251 = Path To String(path=w4921) -> (string=w4935:string)
                n3252 = Build Array(w4916, w4916, w4916, w4916, w4916, w4916, w4916, w4916) -> (w4917:dbl[])
                n3253 = String Length(string=w4935) -> (length=w4934:i32)
                n3254 = Subtract(x=w4934, y=4) -> (x-y=w4932:i32)
                n3255 = Array Size(array=w4917) -> (size(s)=w4919:i32)
                n3256 = String Subset(string=w4935, length (rest)=w4932) -> (substring=w4931:string)  [unwired: 1 out]
                n3257 = To Double Precision Float(number=w4919) -> (double precision float=w4918:dbl)
                n3258 = Concatenate Strings(w4931, "_pos.dat" ("string")) -> (w4929:string)
                n3259 = Build Array (concatenate)(w4918, w4917) -> (w4915:dbl[])
                n3260 = String To Path(string=w4929) -> (path=w4925:path)
                n3261 = Open/Create/Replace File(file path (use dialog)=w4925, operation (0:open)=T25."create", access (0:read/write)=enum16{"read/write", "read-only", "write-only"}."write-only") -> (refnum out=w4926:refnum<file>)  [unwired: 1 in, 4 out]
                n3262 = Deny Access(7:w4926) -> (3:w4922:refnum<file>)  [unwired: 1 in, 2 out]
                n3263 = Write to Binary File(file (use dialog)=w4922, data=w4915, 5:FALSE ("prepend array or string size? (T)"), 9:T24."big-endian, network order" ("byte order (0:big-endian, network order)")) -> (refnum out=w4920:refnum<file>)  [unwired: 1 in, 3 out]
              }
            }
            n3264 = Write to Binary File(file (use dialog)=w4906, data=w4891, 5:w4887, 9:w4885) -> (refnum out=w4888:refnum<file>)  [unwired: 1 in, 3 out]
            n3265 = Write to Binary File(file (use dialog)=w4888, data="Comment (data description)", 5:w4887, 9:w4885) -> (refnum out=w4884:refnum<file>)  [unwired: 1 in, 3 out]
          }
        }
        n3266 = feedback-in #32(w4828) -> ()
        n3267 = feedback-in #33(w4854) -> ()
        n3268 = feedback-in #34(w4827) -> ()
        n3269 = feedback-in #35(w4838) -> ()
        n3270 = feedback-in #36(w4841) -> ()
        n3271 = feedback-in #37(w4853) -> ()
        n3272 = feedback-in #38(w4844) -> ()
      }
      frame #1 {
        n3273 = local read "Saving..."() -> (w5089:bool)
        n3274 = case shown="True" w5089 {
          tunnel: w5093 -> [_ w5105]
          tunnel: w5092 -> [_ w5118]
          tunnel: w5091 -> [_ w5114]
          tunnel: w5090 -> [_ w5113]
          tunnel: w5088 -> [_ w5094]
          tunnel: w5087 -> [_ w5108]
          tunnel: w5086 -> [_ w5107]
          tunnel: w5085 -> [_ w5106]
          tunnel: w5084 -> [_ w5104]
          tunnel: w5083 -> [_ w5102]
          tunnel: w5082 -> [_ w5101]
          tunnel: w5081 -> [_ w5100]
          tunnel: w5080 -> [_ w5099]
          tunnel: w5079 -> [_ w5098]
          tunnel: w5078 -> [_ w5097]
          tunnel: w5077 -> [_ w5096]
          tunnel: w5076 -> [_ w5095]
          frame False {
          }
          frame True {
            n3275 = Multiply(x=w5105, y=w5104) -> (x*y=→"Time (s)":dbl)
            n3276 = Less Or Equal?(x=w5105, y=w5094) -> (x <= y?=w5116:bool)
            n3277 = Or(x="Stop Saving", y="Abort save 2") -> (x .or. y?=w5109:bool)
            n3278 = Not(x=w5109) -> (.not. x?=w5117:bool)
            n3279 = And(x=w5116, y=w5117) -> (x .and. y?=w5115:bool)
            n3280 = case shown="True" w5115 {
              tunnel: w5118 -> [w5126 w5201]
              tunnel: [0.0 w5204] -> w5112
              tunnel: w5105 -> [_ w5202]
              tunnel: w5094 -> [_ w5203]
              tunnel: w5114 -> [_ w5198]
              tunnel: w5113 -> [_ _]
              tunnel: w5108 -> [w5124 w5191]
              tunnel: w5107 -> [w5123 w5192]
              tunnel: w5106 -> [_ w5190]
              tunnel: w5102 -> [_ w5189]
              tunnel: w5101 -> [_ w5133]
              tunnel: w5100 -> [_ w5182]
              tunnel: w5099 -> [_ w5160]
              tunnel: w5098 -> [w5120 w5142]
              tunnel: w5097 -> [w5121 w5141]
              tunnel: w5096 -> [_ w5138]
              tunnel: w5095 -> [_ w5136]
              frame False {
                w5122 = FALSE
                n3281 = Close File(refnum=w5126) -> ()  [unwired: 1 in, 2 out]
                n3282 = case shown="True" w5123 {
                  tunnel: w5124 -> [_ w5128]
                  frame False {
                  }
                  frame True {
                    n3283 = Close File(refnum=w5128) -> ()  [unwired: 1 in, 2 out]
                  }
                }
                n3284 = case shown="True" w5120 {
                  tunnel: w5121 -> [_ w5127]
                  frame False {
                  }
                  frame True {
                    n3285 = Close File(refnum=w5127) -> ()  [unwired: 1 in, 2 out]
                  }
                }
                n3286 = call <vilib>:"Beep.vi"() -> ()  [unwired: 3 in, 9 out]
                n3287 = local write "Raster Scanning..."(w5122) -> ()
                n3288 = local write "Calibrating..."(w5122) -> ()
                n3289 = property on="Abort wiggle" class="Bool (strict)"("Val(Sgnl)"=TRUE) -> ()  [unwired: 2 in, 2 out]
                n3290 = local write "Stop Saving"(w5122) -> ()
                "Saving..." <- w5122
              }
              frame True {
                n3291 = local read "Calibrating..."() -> (w5193:bool)
                n3292 = case "Write fl. data" shown="True" w5192 {
                  tunnel: w5191 -> [_ w5227]
                  tunnel: w5190 -> [_ w5226]
                  frame False {
                  }
                  frame True {
                    n3293 = Write to Binary File(file (use dialog)=w5227, data=w5226, 5:FALSE ("prepend array or string size? (T)"), 9:T24."big-endian, network order" ("byte order (0:big-endian, network order)")) -> ()  [unwired: 1 in, 4 out]
                  }
                }
                n3294 = Greater?(x="Save ave N", y=1.0) -> (0:w5196:bool)
                n3295 = Not(x=w5193) -> (.not. x?=w5195:bool)
                n3296 = And(x=w5195, y=w5196) -> (x .and. y?=w5139:bool)
                n3297 = case shown="True" w5139 {
                  tunnel: w5138 -> [w5207 w5218]
                  tunnel: [w5207 w5210] -> w5137
                  tunnel: "Save ave N" -> [_ w5211]
                  frame False {
                  }
                  frame True {
                    w5208 = 2 ("dimension size")
                    n3298 = Array Size(array=w5218) -> (size(s)=w5212:i32)
                    n3299 = Divide(x=w5212, y=w5208) -> (x/y=w5216:dbl)
                    n3300 = Reshape Array(w5218, w5216, w5208) -> (w5217:u64[][])
                    n3301 = Transpose 2D Array(2D array=w5217) -> (transposed array=w5215:u64[][])
                    n3302 = for {
                      tunnel: w5215 -> [w5220] mode=indexing
                      tunnel: [w5219] -> w5209 mode=indexing
                      tunnel: w5211 -> [w5221]
                      workers-P: _ -> [_]
                      n3303 = call "downsample 1D array - U64.vi"("Ave N"=w5221, "Array In"=w5220) -> ("Array Out"=w5219:u64[])  [unwired: 1 in]
                    }
                    n3304 = Transpose 2D Array(2D array=w5209) -> (transposed array=w5214:u64[][])
                    n3305 = Divide(x=w5212, y=w5211) -> (x/y=w5213:dbl)
                    n3306 = Reshape Array(w5214, w5213) -> (w5210:u64[])
                  }
                }
                n3307 = case shown="True" w5139 {
                  tunnel: w5198 -> [w5230 w5242]
                  tunnel: [w5230 w5234] -> w5194
                  tunnel: "Save ave N" -> [_ w5235]
                  tunnel: w5189 -> [_ w5233]
                  frame False {
                  }
                  frame True {
                    n3308 = Array Size(array=w5242) -> (size(s)=w5236:i32)
                    n3309 = Array Size(array=w5233) -> (size(s)=w5232:i32)
                    n3310 = Divide(x=w5236, y=w5232) -> (x/y=w5240:dbl)
                    n3311 = Reshape Array(w5242, w5240, w5232) -> (w5241:i16[][])
                    n3312 = Transpose 2D Array(2D array=w5241) -> (transposed array=w5239:i16[][])
                    n3313 = for {
                      tunnel: w5239 -> [w5245] mode=indexing
                      tunnel: [w5244] -> w5231 mode=indexing
                      tunnel: w5235 -> [w5243]
                      workers-P: _ -> [_]
                      n3314 = call "downsample 1D array - I16.vi"("Ave N"=w5243, "Array In"=w5245) -> ("Array Out"=w5244:i16[])  [unwired: 1 out]
                    }
                    n3315 = Transpose 2D Array(2D array=w5231) -> (transposed array=w5238:i16[][])
                    n3316 = Divide(x=w5236, y=w5235) -> (x/y=w5237:dbl)
                    n3317 = Reshape Array(w5238, w5237) -> (w5234:i16[])
                  }
                }
                n3318 = Index Array(array=w5160, index=1) -> (element=w5163:waveform(dbl))
                n3319 = Index Array(array=w5160, index=0) -> (element=w5165:waveform(dbl))
                n3320 = Unbundle By Name(w5163) -> ("Y"=w5167:dbl[])
                n3321 = Unbundle By Name(w5165) -> ("Y"=w5175:dbl[])
                n3322 = case "Write trap pos. data" shown="True" w5142 {
                  tunnel: w5141 -> [_ w5223]
                  tunnel: w5137 -> [_ w5222]
                  frame False {
                  }
                  frame True {
                    n3323 = Write to Binary File(file (use dialog)=w5223, data=w5222, 5:FALSE ("prepend array or string size? (T)"), 9:T24."big-endian, network order" ("byte order (0:big-endian, network order)")) -> ()  [unwired: 1 in, 4 out]
                  }
                }
                n3324 = Write to Binary File(file (use dialog)=w5201, data=w5194, 5:FALSE ("prepend array or string size? (T)"), 9:T24."big-endian, network order" ("byte order (0:big-endian, network order)")) -> ()  [unwired: 1 in, 4 out]
                n3325 = feedback #39(w5167) -> (w5169:dbl[])
                n3326 = Build Array (concatenate)(w5169, w5167) -> (w5168:dbl[])
                n3327 = Select(t=w5167, s=w5133, f=w5168) -> (s? t:f=w5153:dbl[])
                n3328 = feedback-in #39(w5153) -> ()
                n3329 = feedback #40(w5175) -> (w5188:dbl[])
